vi "IK Solver.vi"() -> ()   [LabVIEW 2024]
uses:
  <vilib>/Utility/miscctls.llb/LV3DPointTypeDef.ctl
  <vilib>/Analysis/_algsub.llb/Real PseudoInverse Matrix.vi
  <vilib>/Analysis/baseanly.llb/A x Vector.vi
  <vilib>/Analysis/NI_AALBase.lvlib
  <vilib>/Analysis/NI_AALPro.lvlib
  <vilib>/Analysis/Matrix/Datatypes/RealMatrix.ctl
  <vilib>/Analysis/Matrix/NI_Matrix.lvlib
panel:
  out "error":dbl[](array[numeric])
  out "3D Picture":refnum<vi>(3d-picture)
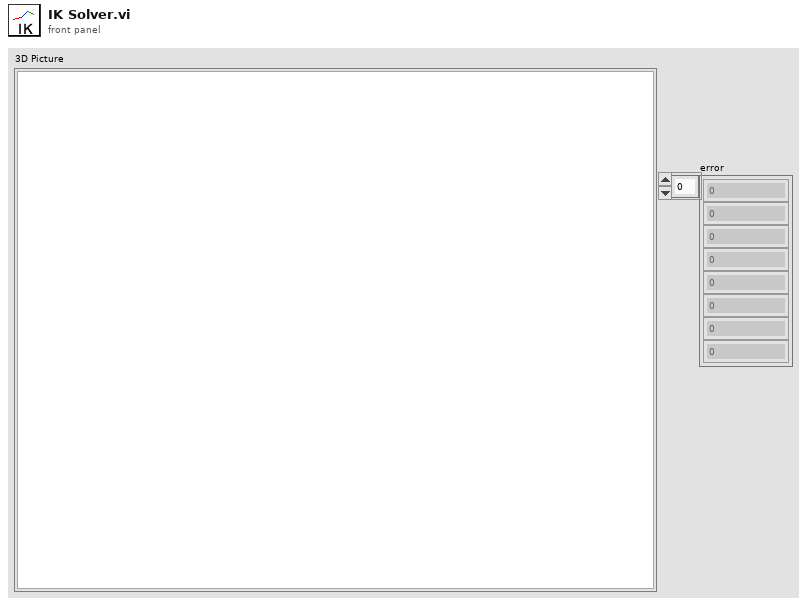
[diagram p1: front panel]
types:
  T1 = cluster{"Theta (degrees)":dbl, "d":dbl, "a":dbl, "alpha (degrees)":dbl}[]
  T2 = typedef "LV3DPointTypeDef.ctl" = cluster{"X":sgl, "Y":sgl, "Z":sgl}
  T3 = typedef "NI_Matrix.lvlib/RealMatrix.ctl" = dbl[][]
  T4 = cluster{"Theta (degrees)":dbl, "d":dbl, "a":dbl, "alpha (degrees)":dbl}
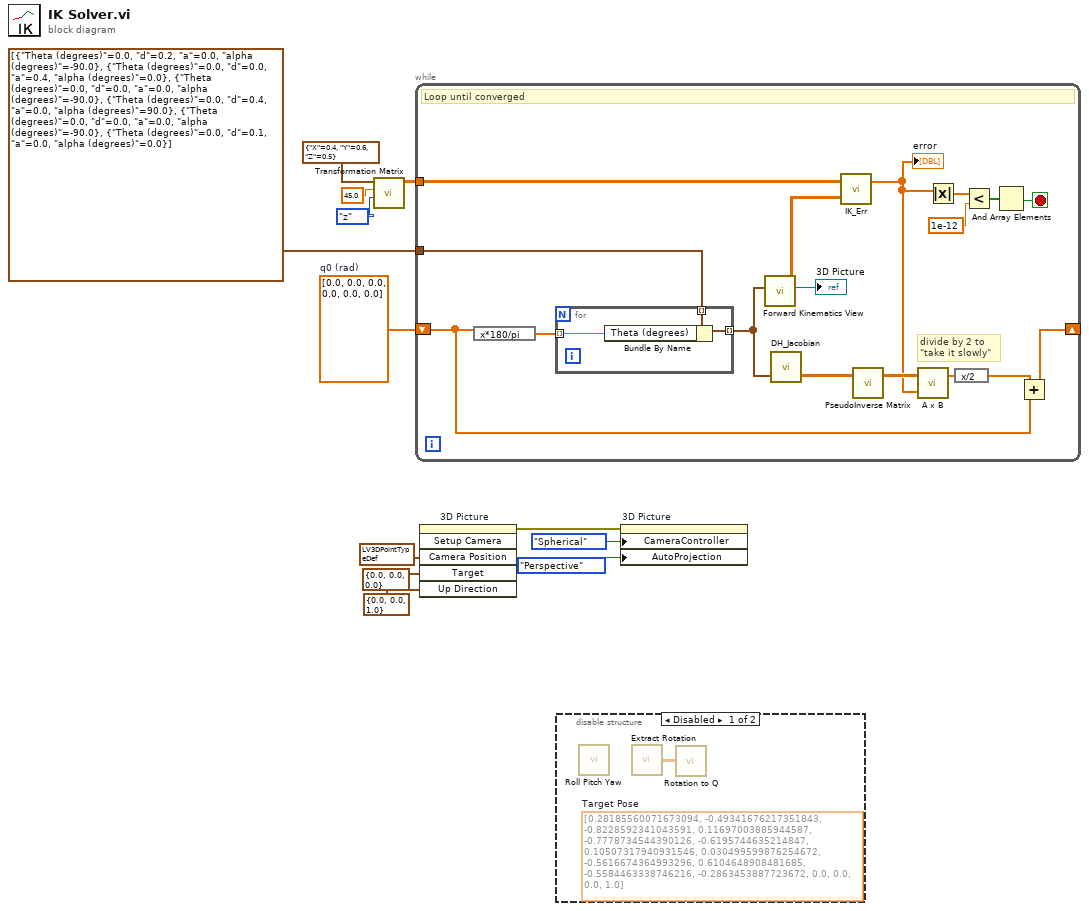
[diagram p0: block diagram]
diagram:
  w5 = sgl[] [0.0, 0.0, 0.0, 0.0, 0.0, 0.0]  # q0 (rad)
  n1 = call <userlib>:"Transformation Matrix.vi"("Axis"=enum16{"x", "y", "z"}."z", "Angle (degrees)"=45.0, "Translation"=cluster{"X":dbl, "Y":dbl, "Z":dbl} {"X"=0.4, "Y"=0.6, "Z"=0.5}) -> ("Transformation Matrix"=w1:T3)  [unwired: 8 in]
  n2 = while {
    shift-right: [w24] -> _
    shift-left: w5 -> [w25]
    tunnel: T1 [{"Theta (degrees)"=0.0, "d"=0.2, "a"=0.0, "alpha (degrees)"=-90.0}, {"Theta (degrees)"=0.0, "d"=0.0, "a"=0.4, "alpha (degrees)"=0.0}, {"Theta (degrees)"=0.0, "d"=0.0, "a"=0.0, "alpha (degrees)"=-90.0}, {"Theta (degrees)"=0.0, "d"=0.4, "a"=0.0, "alpha (degrees)"=90.0}, {"Theta (degrees)"=0.0, "d"=0.0, "a"=0.0, "alpha (degrees)"=-90.0}, {"Theta (degrees)"=0.0, "d"=0.1, "a"=0.0, "alpha (degrees)"=0.0}] -> [w14]
    tunnel: w1 -> [w13]
    stop <- w15 stop-if-true
    # "divide by 2 to \n\"take it slowly\""
    # "Loop until converged"
    n3 = expression code="x*180/pi"(w25) -> (w28:dbl[])
    n4 = for {
      tunnel: w14 -> [w32] mode=indexing
      tunnel: w28 -> [w31] mode=indexing
      tunnel: [w30] -> w27 mode=indexing
      n5 = Bundle By Name(cluster=w32, "Theta (degrees)"=w31) -> (w30:T4)
    }
    n6 = call <userlib>:"Forward Kinematics View.vi"("Joints"=w27) -> ("3D Picture"=→"3D Picture":refnum<vi>, "end effector pose"=w21:T3)  [unwired: 9 in]
    n7 = call <userlib>:"DH_Jacobian.vi"("Joints"=w27) -> ("Jacobian"=w23:dbl[][])  [unwired: 1 in, 1 out]
    n8 = call <userlib>:"IK_Err.vi"("end effector pose"=w21, "Target Pose"=w13) -> ("error"=w17:dbl[])  [unwired: 1 in]
    "error" <- w17
    n9 = call-poly <vilib>:"PseudoInverse Matrix.vi"("Input Matrix"=w23) -> ("PseudoInverse Matrix"=w22:T3)  [unwired: 1 in, 1 out]
    n10 = call-poly <vilib>:"A x B.vi"("Vector"=w17, "A"=w22) -> ("A x Vector"=w26:dbl[])  [unwired: 1 out]
    n11 = Absolute Value(x=w17) -> (abs(x)=w18:dbl[])
    n12 = expression code="x/2"(w26) -> (w16:dbl[])
    n13 = Less?(x=w18, y=1e-12) -> (x < y?=w20:bool[])
    n14 = And Array Elements(Boolean array=w20) -> (logical AND=w15:bool)
    n15 = Add(x=w16, y=w25) -> (x+y=w24:dbl[])
  }
  n16 = invoke on="3D Picture" class="SceneGraphDisp (strict)" method="Setup Camera"("Camera Position"=T2 {"X"=2.0, "Y"=2.0, "Z"=0.1}, "Target"=cluster{"X":sgl, "Y":sgl, "Z":sgl} {"X"=0.0, "Y"=0.0, "Z"=0.0}, "Up Direction"=cluster{"X":sgl, "Y":sgl, "Z":sgl} {"X"=0.0, "Y"=0.0, "Z"=1.0}) -> (error out=w12:errorcluster)  [unwired: 3 in, 5 out]
  n17 = disable-structure shown="Disabled" {
    frame Disabled {
      (unwired) T3 [[0.28185560071673094, -0.49341676217351843, -0.8228592341043591, 0.11697003885944587], [-0.7778734544390126, -0.6195744635214847, 0.10507317940931546, 0.030499599876254672], [-0.5616674364993296, 0.6104648908481685, -0.5584463338746216, -0.2863453887723672], [0.0, 0.0, 0.0, 1.0]]  # Target Pose
      n18 = call <userlib>:"Roll Pitch Yaw.vi"() -> ()  [unwired: 1 in, 1 out]
      n19 = call <userlib>:"Extract Rotation.vi"() -> ("Rotation matrix"=w33:T3)  [unwired: 1 in]
      n20 = call <userlib>:"Rotation to Q.vi"("Rotation matrix"=w33) -> ()  [unwired: 1 out]
    }
    frame Enabled {
    }
  }
  n21 = property on="3D Picture" class="SceneGraphDisp (strict)"(error in=w12, "CameraController"=enum16{"None", "Spherical", "Flying"}."Spherical" ("Camera Controller"), "AutoProjection"=enum16{"None", "Perspective", "Orthographic"}."Perspective" ("Auto Projection Mode")) -> ()  [unwired: 1 in, 2 out]
